vi "subvi_Counter.vi"(8 "error in (no error)":errorcluster, 11 "Reset?":bool) -> (0 "error out":errorcluster, 3 "Counter (I32)":i32)   [LabVIEW 2015, in "File Version Lib.lvlib"]
uses:
  File Version Lib.lvlib
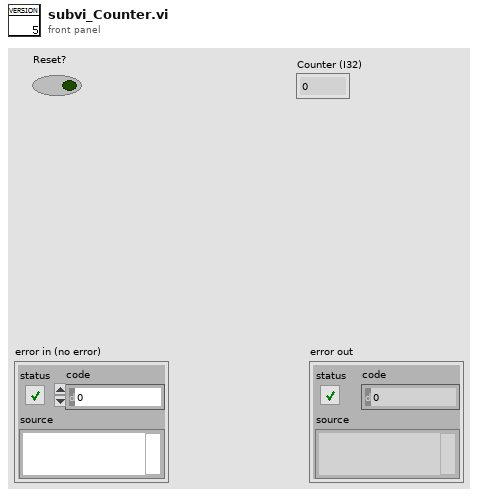
[diagram p1: front panel]
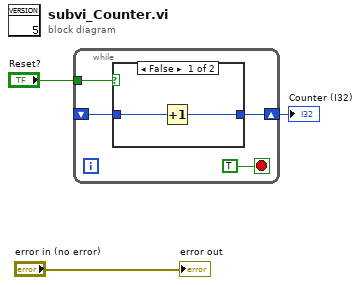
[diagram p0: block diagram]
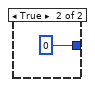
[diagram p2: hidden frame]
diagram:
  n1 = while {
    shift-right: [w7] -> w2
    shift-left: _ -> [w6]
    tunnel: "Reset?" -> [w4]
    stop <- TRUE stop-if-true
    n2 = case shown="False" w4 {
      tunnel: [w9 0] -> w7
      tunnel: w6 -> [w8 _]
      frame False {
        n3 = Increment(x=w8) -> (x+1=w9:i32)
      }
      frame True {
      }
    }
  }
  "Counter (I32)" <- w2
  "error out" <- "error in (no error)"
